vi "TCP Multiple Connections - Client 1.vi"() -> ()   [LabVIEW 2015]
doc: "Establishes a connection to TCP Multiple Connections - Server.vi. After you click the Stop button, this VI sends a single character to tell the Server VI to terminate the connection."
panel:
  in  "Server Closed":string="The server VI closed the connection."
  out "Data from Server":dbl(graph)
  in  "Stop":bool
  # "Overview: Demonstrates the use of the TCP functions to connect to a TCP server VI that is sending data to multiple client VIs.\nInstructions:\n1. Ensure TCP Multiple Connections - Server.vi is already running.\n2. Run the VI.\n3. Note that the Data from Server chart starts updating, and the Number of Client Connections value on the server VI increments by 1.\n4. Click Stop to stop the VI. Note that the Number of Client Connections value on the server VI decrements by 1."
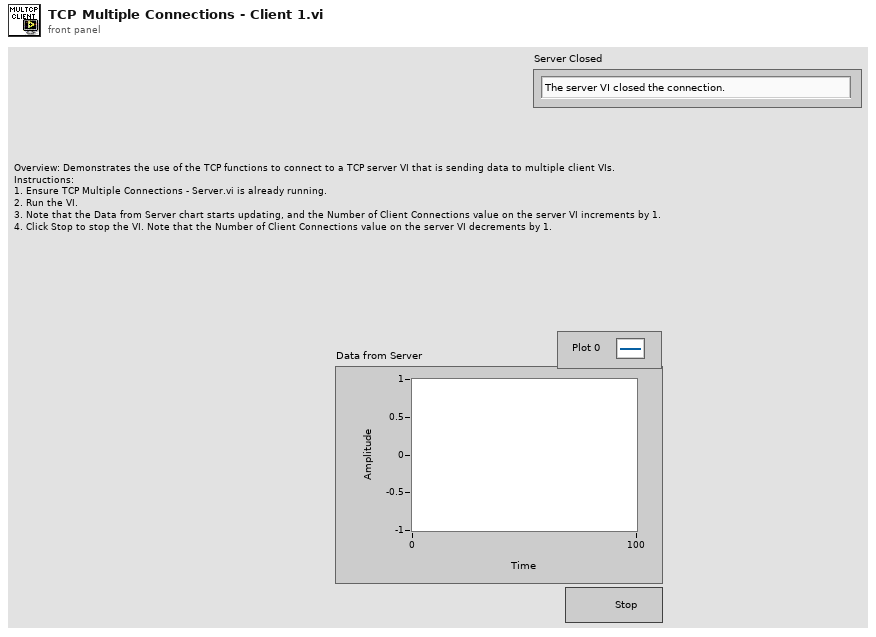
[diagram p1: front panel]
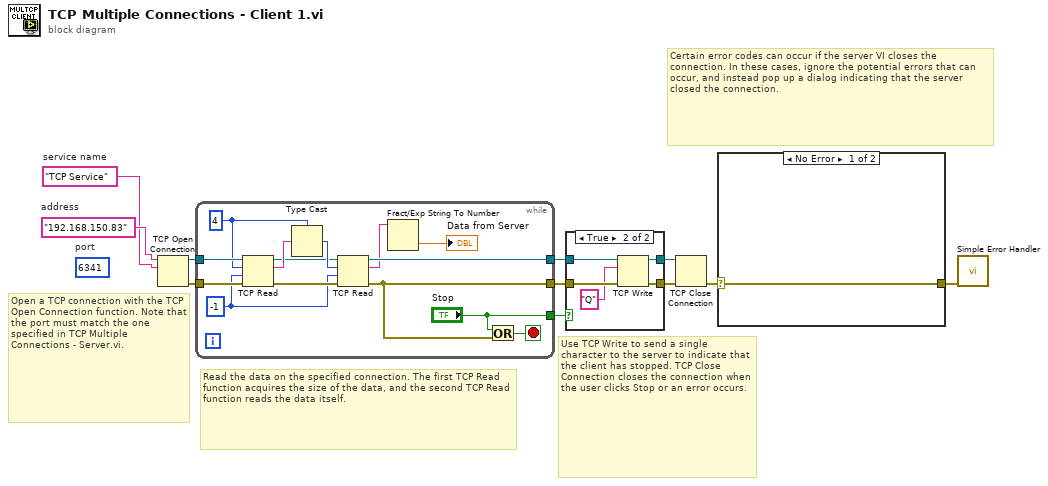
[diagram p0: block diagram]
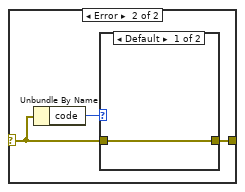
[diagram p2: hidden frame]
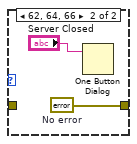
[diagram p3: hidden frame]
diagram:
  w1 = "TCP Service"  # service name
  (unwired) u16 6341  # port
  w2 = "192.168.150.83"  # address
  # "Certain error codes can occur if the server VI closes the connection. In these cases, ignore the potential errors that can occur, and instead pop up a dialog indicating that the server closed the connection."
  # "Use TCP Write to send a single character to the server to indicate that the client has stopped. TCP Close Connection closes the connection when the user clicks Stop or an error occurs."
  # "Read the data on the specified connection. The first TCP Read function acquires the size of the data, and the second TCP Read function reads the data itself."
  # "Open a TCP connection with the TCP Open Connection function. Note that the port must match the one specified in TCP Multiple Connections - Server.vi."
  n1 = TCP Open Connection(address=w2, remote port or service name=w1) -> (connection ID=w11:refnum<k5>, error out=w10:errorcluster)  [unwired: 1 in, 2 out]
  n2 = while {
    tunnel: ["Stop"] -> w5
    tunnel: [w19] -> w9
    tunnel: [w16] -> w7
    tunnel: w10 -> [w24]
    tunnel: w11 -> [w25]
    stop <- w18 stop-if-true
    w12 = -1
    w13 = 4
    n3 = TCP Read(connection ID=w25, bytes to read=w13, error in (no error)=w24, 9:w12) -> (connection ID out=w20:refnum<k5>, data out=w23:string, error out=w22:errorcluster)  [unwired: 1 out]
    n4 = Type Cast(type=w13, x=w23) -> (*(type *) &x=w21:i32)
    n5 = TCP Read(connection ID=w20, bytes to read=w21, error in (no error)=w22, 9:w12) -> (connection ID out=w19:refnum<k5>, data out=w15:string, error out=w16:errorcluster)  [unwired: 1 out]
    n6 = Fract/Exp String To Number(string=w15) -> (number=→"Data from Server":dbl)  [unwired: 3 in, 1 out]
    n7 = Or(x="Stop", y=w16) -> (x .or. y?=w18:bool)
  }
  n8 = case shown="True" w5 {
    tunnel: w9 -> [w27 w32]
    tunnel: [w27 w30] -> w8
    tunnel: w7 -> [w26 w31]
    tunnel: [w26 w29] -> w6
    frame False {
    }
    frame True {
      n9 = TCP Write(connection ID=w32, data in="Q", error in (no error)=w31) -> (connection ID out=w30:refnum<k5>, error out=w29:errorcluster)  [unwired: 2 out]
    }
  }
  n10 = TCP Close Connection(connection ID=w8, error in (no error)=w6) -> (error out=w4:errorcluster)  [unwired: 2 out]
  n11 = case shown="No Error" w4 {
    selector: w4 -> [w33 w35]
    tunnel: [w33 w34] -> w3
    frame No Error {
    }
    frame Error {
      n12 = Unbundle By Name(w35) -> ("code"=w36:i32)
      n13 = case shown="Default" w36 {
        tunnel: w35 -> [w37 _]
        tunnel: [w37 w39] -> w34
        frame Default {
        }
        frame 62, 64, 66 {
          w39 = errorcluster {"status"=FALSE, "code"=0, "source"=""}  # No error
          n14 = One Button Dialog(message="Server Closed") -> ()  [unwired: 1 in, 1 out]
        }
      }
    }
  }
  n15 = call <vilib>:"Simple Error Handler.vi"("error in (no error)"=w3) -> ()  [unwired: 1 in, 8 out]
